vi "FGV_timer_frec_G01.vi"(7 "Action":T1=enum."Get Time", 8 "error in (no error)":errorcluster, 11 "Target Time":dbl) -> (0 "error out":errorcluster, 2 "time elapsed?":bool, 3 "elapsed time":dbl)   [LabVIEW 2018]
uses:
  Controls/FGV_savetime_action.ctl
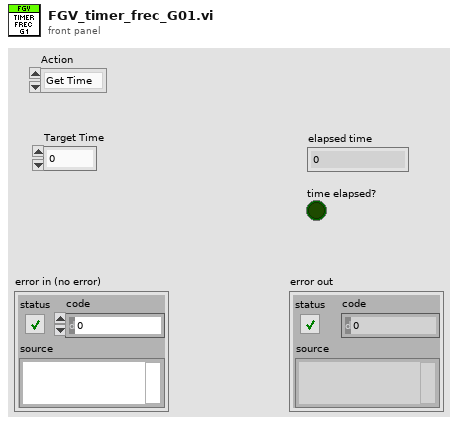
[diagram p1: front panel]
types:
  T1 = typedef "FGV_savetime_action.ctl" = enum16{"Start Timer", "Get Time"}
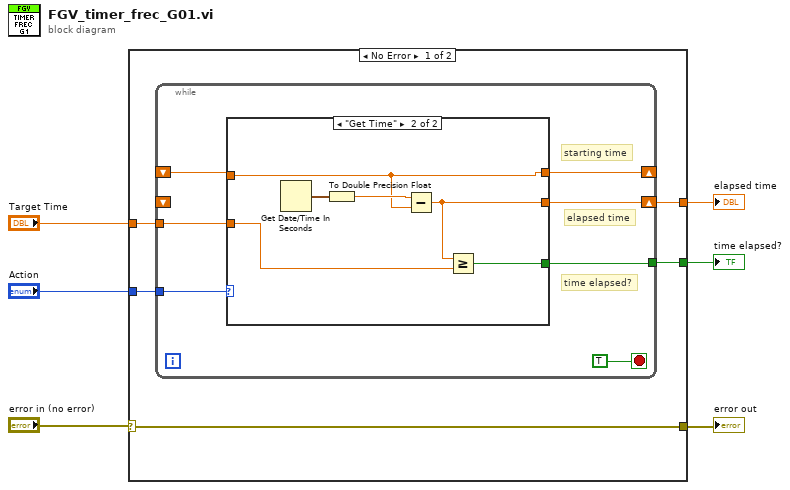
[diagram p0: block diagram]
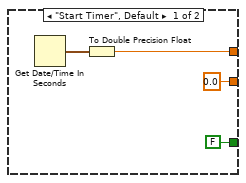
[diagram p2: hidden frame]
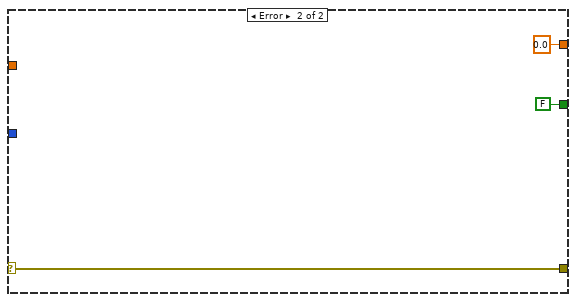
[diagram p3: hidden frame]
diagram:
  n1 = case shown="No Error" "error in (no error)" {
    selector: "error in (no error)" -> [w7 w31]
    tunnel: "Action" -> [w11 _]
    tunnel: "Target Time" -> [w10 _]
    tunnel: [w9 FALSE] -> w4
    tunnel: [w8 0.0] -> w3
    tunnel: [w7 w31] -> w1
    frame No Error {
      n2 = while {
        tunnel: w11 -> [w17]
        shift-right: [w16] -> w8
        shift-left: _ -> [_]
        tunnel: w10 -> [w15]
        tunnel: [w14] -> w9
        shift-right: [w13] -> _
        shift-left: _ -> [w12]
        stop <- TRUE stop-if-true
        # "starting time"
        # "time elapsed?"
        # "elapsed time"
        n3 = case shown="\"Get Time\"" w17 {
          tunnel: w12 -> [_ w23]
          tunnel: [0.0 w28] -> w16
          tunnel: w15 -> [_ w27]
          tunnel: [FALSE w26] -> w14
          tunnel: [w20 w23] -> w13
          frame "Start Timer", Default {
            n4 = Get Date/Time In Seconds() -> (seconds since 1Jan1904=w21:timestamp)
            n5 = To Double Precision Float(number=w21) -> (double precision float=w20:dbl)
          }
          frame "Get Time" {
            n6 = Get Date/Time In Seconds() -> (seconds since 1Jan1904=w25:timestamp)
            n7 = To Double Precision Float(number=w25) -> (double precision float=w24:dbl)
            n8 = Subtract(x=w24, y=w23) -> (x-y=w28:dbl)
            n9 = Greater Or Equal?(x=w28, y=w27) -> (x >= y?=w26:bool)
          }
        }
      }
    }
    frame Error {
    }
  }
  "time elapsed?" <- w4
  "elapsed time" <- w3
  "error out" <- w1
